vi "ADC sample.vi"(11 "error in (no error)":errorcluster) -> (15 "error out":errorcluster)   [LabVIEW 2012]
doc: "This example starts and runs a bulk ADC read."
uses:
  Controls/ADC_Setconfig.ctl
  Controls/Gain Mode.ctl
  Controls/Calibration Mode.ctl
  Controls/Bulk Wrapper Action.ctl
panel:
  in  "Live display?":bool
  out "Acquired Data":dbl[][](graph) caption="pBuf 3"
  out "Actual Frequency (Hz)":dbl=1000.0
  in  "Samples to be taken":u32=1000
  in  "Output Frequency (Hz)":dbl=1000.0
  out "BytesLeft":u32
  in  "stop":bool caption="stop 2"
  in  "Trigger & Counter bits":T1={"Timer Trigger"=TRUE, "External Tigger"=FALSE, "Scan"=TRUE, "Falling Edge"=FALSE, "CRT0 Ext"=FALSE}
  in  "DeviceIndex":u32
  in  "Oversamples":u8
  in  "End Channel":u8=15
  in  "Start Channel":u8
  in  "Channels":T2=[{"Gain Mode"=enum."+/- 10V", "Differential Mode"=FALSE}, {"Gain Mode"=enum."+/- 10V", "Differential Mode"=FALSE}, {"Gain Mode"=enum."+/- 10V", "Differential Mode"=FALSE}, {"Gain Mode"=enum."+/- 10V", "Differential Mode"=FALSE}, {"Gain Mode"=enum."+/- 10V", "Differential Mode"=FALSE}, {"Gain Mode"=enum."+/- 10V", "Differential Mode"=FALSE}, {"Gain Mode"=enum."+/- 10V", "Differential Mode"=FALSE}, {"Gain Mode"=enum."+/- 10V", "Differential Mode"=FALSE}, {"Gain Mode"=enum."+/- 10V", "Differential Mode"=FALSE}, {"Gain Mode"=enum."+/- 10V", "Differential Mode"=FALSE}, {"Gain Mode"=enum."+/- 10V", "Differential Mode"=FALSE}, {"Gain Mode"=enum."+/- 10V", "Differential Mode"=FALSE}, {"Gain Mode"=enum."+/- 10V", "Differential Mode"=FALSE}, {"Gain Mode"=enum."+/- 10V", "Differential Mode"=FALSE}, {"Gain Mode"=enum."+/- 10V", "Differential Mode"=FALSE}, {"Gain Mode"=enum."+/- 10V", "Differential Mode"=FALSE}] caption="Channels (Scroll down to set all active channels)"
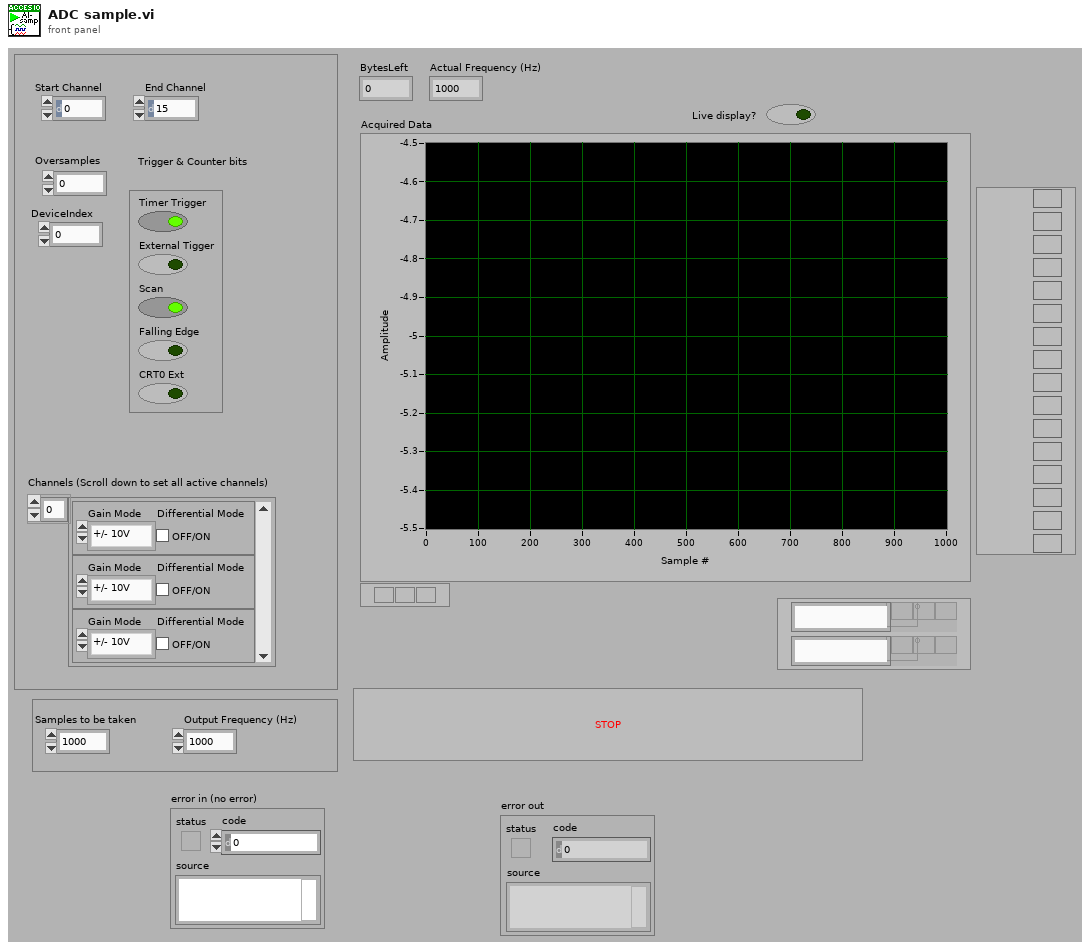
[diagram p1: front panel]
types:
  T1 = cluster{"Timer Trigger":bool, "External Tigger":bool, "Scan":bool, "Falling Edge":bool, "CRT0 Ext":bool}
  T2 = typedef "ADC_Setconfig.ctl" = cluster{"Gain Mode":T3, "Differential Mode":bool}[]
  T3 = typedef "Gain Mode.ctl" = enum8{"0-10V", "+/- 10V", "0-5V", "+/- 5V", "0-2V", "+/- 2V", "0-1V", "+/- 1V"}
  T4 = typedef "Calibration Mode.ctl" = enum8{"Acquire Data", "Acquire Ground", "Do not use", "Aquire Cal. Ref."}
  T5 = cluster{"Gain Mode":T3, "Differential Mode":bool}
  T6 = typedef "Bulk Wrapper Action.ctl" = enum16{"Start Read", "Read Buffer"}
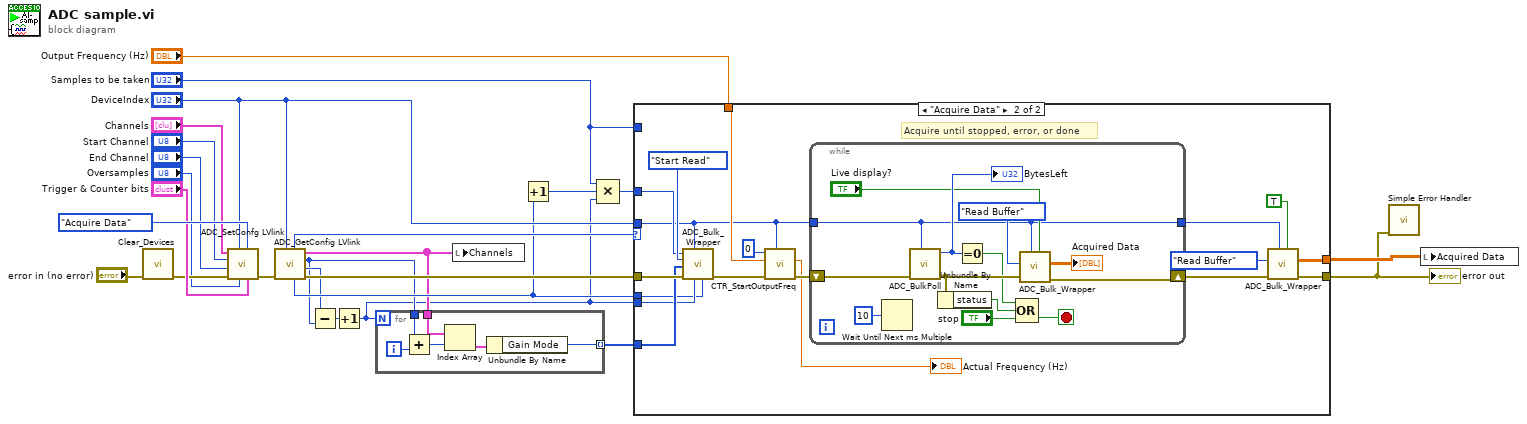
[diagram p0: block diagram]
diagram:
  n1 = call "Clear_Devices.vi"("error in (no error)"="error in (no error)") -> ("error out"=w21:errorcluster)  [unwired: 10 in]
  n2 = call "ADC_SetConfg LVlink.vi"("Trigger & Counter bits"="Trigger & Counter bits", "Calibration Mode"=Calibration_Mode."Acquire Data", "Oversamples"="Oversamples", "DeviceIndex"="DeviceIndex", "error in (no error)"=w21, "End Channel"="End Channel", "Start Channel"="Start Channel", "Channels"="Channels") -> ("error out"=w19:errorcluster)  [unwired: 3 in]
  n3 = call "ADC_GetConfig LVlink.vi"("DeviceIndex"="DeviceIndex", "error in (no error)"=w19) -> ("error out"=w18:errorcluster, "End Channel"=w6:u8, "Start Channel"=w4:u8, "Channels"=w3:T2, "Oversamples"=w7:u8, "Calibration Mode"=w9:T4)  [unwired: 3 in, 1 out]
  n4 = Subtract(x=w6, y=w4) -> (x-y=w5:u8)
  n5 = Increment(x=w5) -> (x+1=w2:u8)
  n6 = for {
    N: w2 -> [_]
    tunnel: w3 -> [w28]
    tunnel: [w31] -> w13 mode=indexing
    tunnel: w4 -> [w29]
    i -> [w30]
    n7 = Add(x=w29, y=w30) -> (x+y=w26:i32)
    n8 = Index Array(array=w28, index=w26) -> (element=w27:T5)
    n9 = Unbundle By Name(w27) -> ("Gain Mode"=w31:T3)
  }
  n10 = local write "Channels"(w3) -> ()
  n11 = Increment(x=w7) -> (x+1=w8:u8)
  n12 = Compound Arithmetic op=MULTIPLY("Samples to be taken", w8, w2) -> (w20:u32)
  n13 = case shown="\"Acquire Data\"" w9 {
    tunnel: w20 -> [_ w49]
    tunnel: w7 -> [_ w45]
    tunnel: w2 -> [_ w46]
    tunnel: w18 -> [w32 w48]
    tunnel: "DeviceIndex" -> [_ w34]
    tunnel: "Samples to be taken" -> [_ _]
    tunnel: w13 -> [_ w47]
    tunnel: "Output Frequency (Hz)" -> [_ w35]
    tunnel: [w32 w40] -> w10
    tunnel: [_ w39] -> w11
    frame Default {
    }
    frame "Acquire Data" {
      # "Acquire until stopped, error, or done"
      n14 = call "ADC_Bulk_Wrapper.vi"("oversamples"=w45, "# channels"=w46, "DeviceIndex"=w34, "error in (no error)"=w48, "Gains In"=w47, "Action"=Bulk_Wrapper_Action."Start Read" ("Enum"), "BufSize(32bit samples)"=w49) -> ("error out"=w37:errorcluster)  [unwired: 1 in, 3 out]
      n15 = call "CTR_StartOutputFreq.vi"("DeviceIndex"=w34, "error in (no error)"=w37, "Output Frequency (Hz)"=w35, "BlockIndex"=u32 0) -> ("error out"=w36:errorcluster, "Actual Frequency (Hz)"=→"Actual Frequency (Hz)":dbl)  [unwired: 6 in]
      n16 = while {
        tunnel: w34 -> [w55]
        shift-right: [w58] -> w44
        shift-left: w36 -> [w51]
        tunnel: [w55] -> w43
        stop <- w63 stop-if-true
        n17 = Wait Until Next ms Multiple(millisecond multiple=u32 10) -> ()  [unwired: 1 out]
        n18 = call "ADC_BulkPoll.vi"("DeviceIndex"=w55, "error in (no error)"=w51) -> ("error out"=w59:errorcluster, "BytesLeft"=w61:u32)  [unwired: 8 in]
        "BytesLeft" <- w61
        n19 = Unbundle By Name(w59) -> ("status"=w54:bool)
        n20 = Equal To 0?(x=w61) -> (x = 0?=w53:bool)
        n21 = Compound Arithmetic op=OR(w53, w54, "stop") -> (w63:bool)
        n22 = call "ADC_Bulk_Wrapper.vi"("Process Data?"="Live display?", "DeviceIndex"=w55, "error in (no error)"=w59, "Action"=Bulk_Wrapper_Action."Read Buffer" ("Enum")) -> ("error out"=w58:errorcluster, "Data"=→"Acquired Data":dbl[][])  [unwired: 4 in, 2 out]
      }
      n23 = call "ADC_Bulk_Wrapper.vi"("Process Data?"=TRUE, "DeviceIndex"=w43, "error in (no error)"=w44, "Action"=Bulk_Wrapper_Action."Read Buffer" ("Enum")) -> ("error out"=w40:errorcluster, "Data"=w39:dbl[][])  [unwired: 4 in, 2 out]
    }
  }
  "error out" <- w10
  n24 = call <vilib>:"Simple Error Handler.vi"("error in (no error)"=w10) -> ()  [unwired: 4 in, 5 out]
  n25 = local write "Acquired Data"(w11) -> ()
